vi "Enqueuer.vi"() -> ()   [LabVIEW 2020]
panel:
  out "Tank":dbl(slide) scale=0.0..100.0
  in  "stop":bool
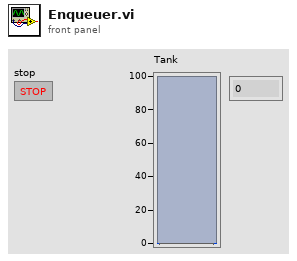
[diagram p1: front panel]
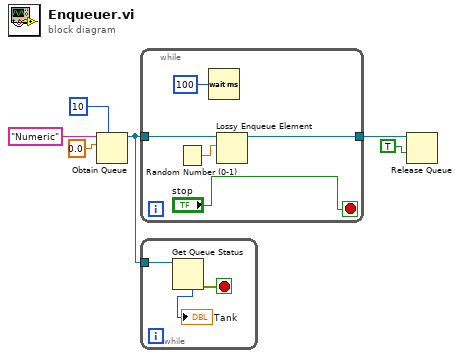
[diagram p0: block diagram]
diagram:
  n1 = Obtain Queue(max queue size (-1, unlimited)=10, name (unnamed)="Numeric", element data type=0.0) -> (queue out=w2:refnum<queue>)  [unwired: 2 in, 2 out]
  n2 = while {
    tunnel: w2 -> [w11]
    tunnel: [w7] -> w4
    stop <- "stop" stop-if-true
    n3 = Random Number (0-1)() -> (number: 0 to 1=w10:dbl)
    n4 = Wait (ms)(milliseconds to wait=u32 100) -> ()  [unwired: 1 out]
    n5 = Lossy Enqueue Element(queue=w11, element=w10) -> (queue out=w7:refnum<queue>)  [unwired: 1 in, 3 out]
  }
  n6 = while {
    tunnel: w2 -> [w13]
    stop <- w14 stop-if-true
    n7 = Get Queue Status(queue=w13) -> (error out=w14:errorcluster, # elements in queue=→"Tank":i32)  [unwired: 2 in, 6 out]
  }
  n8 = Release Queue(queue=w4, force destroy? (F)=TRUE) -> ()  [unwired: 1 in, 3 out]
